vi "Lectura OSA (1).vi"() -> ()   [LabVIEW 2014]
panel:
  out "Read Data":string
  out "Respuesta OSA":string
  out "error out":errorcluster
  out "Array Data":dbl[](array[numeric]) format="%.5e"
  in  "Get data":bool
  in  "Send":bool
  out "Espectro":cluster{dbl[], dbl[]}(graph)
  out "?":bool
  in  "Sweep repeat":bool
  in  "Blank/Disp":bool=TRUE
  in  "?":bool
  in  "Stop":dbl=1570.0
  in  "Start":dbl=1470.0
  in  "Atributo":i32(listbox)
  in  "Trace":i32(listbox)
  in  "Preconfigurar":bool
  in  "Puerto":refnum<visa-resource-name>
  # "Sí"
  # "No"
  # "Span"
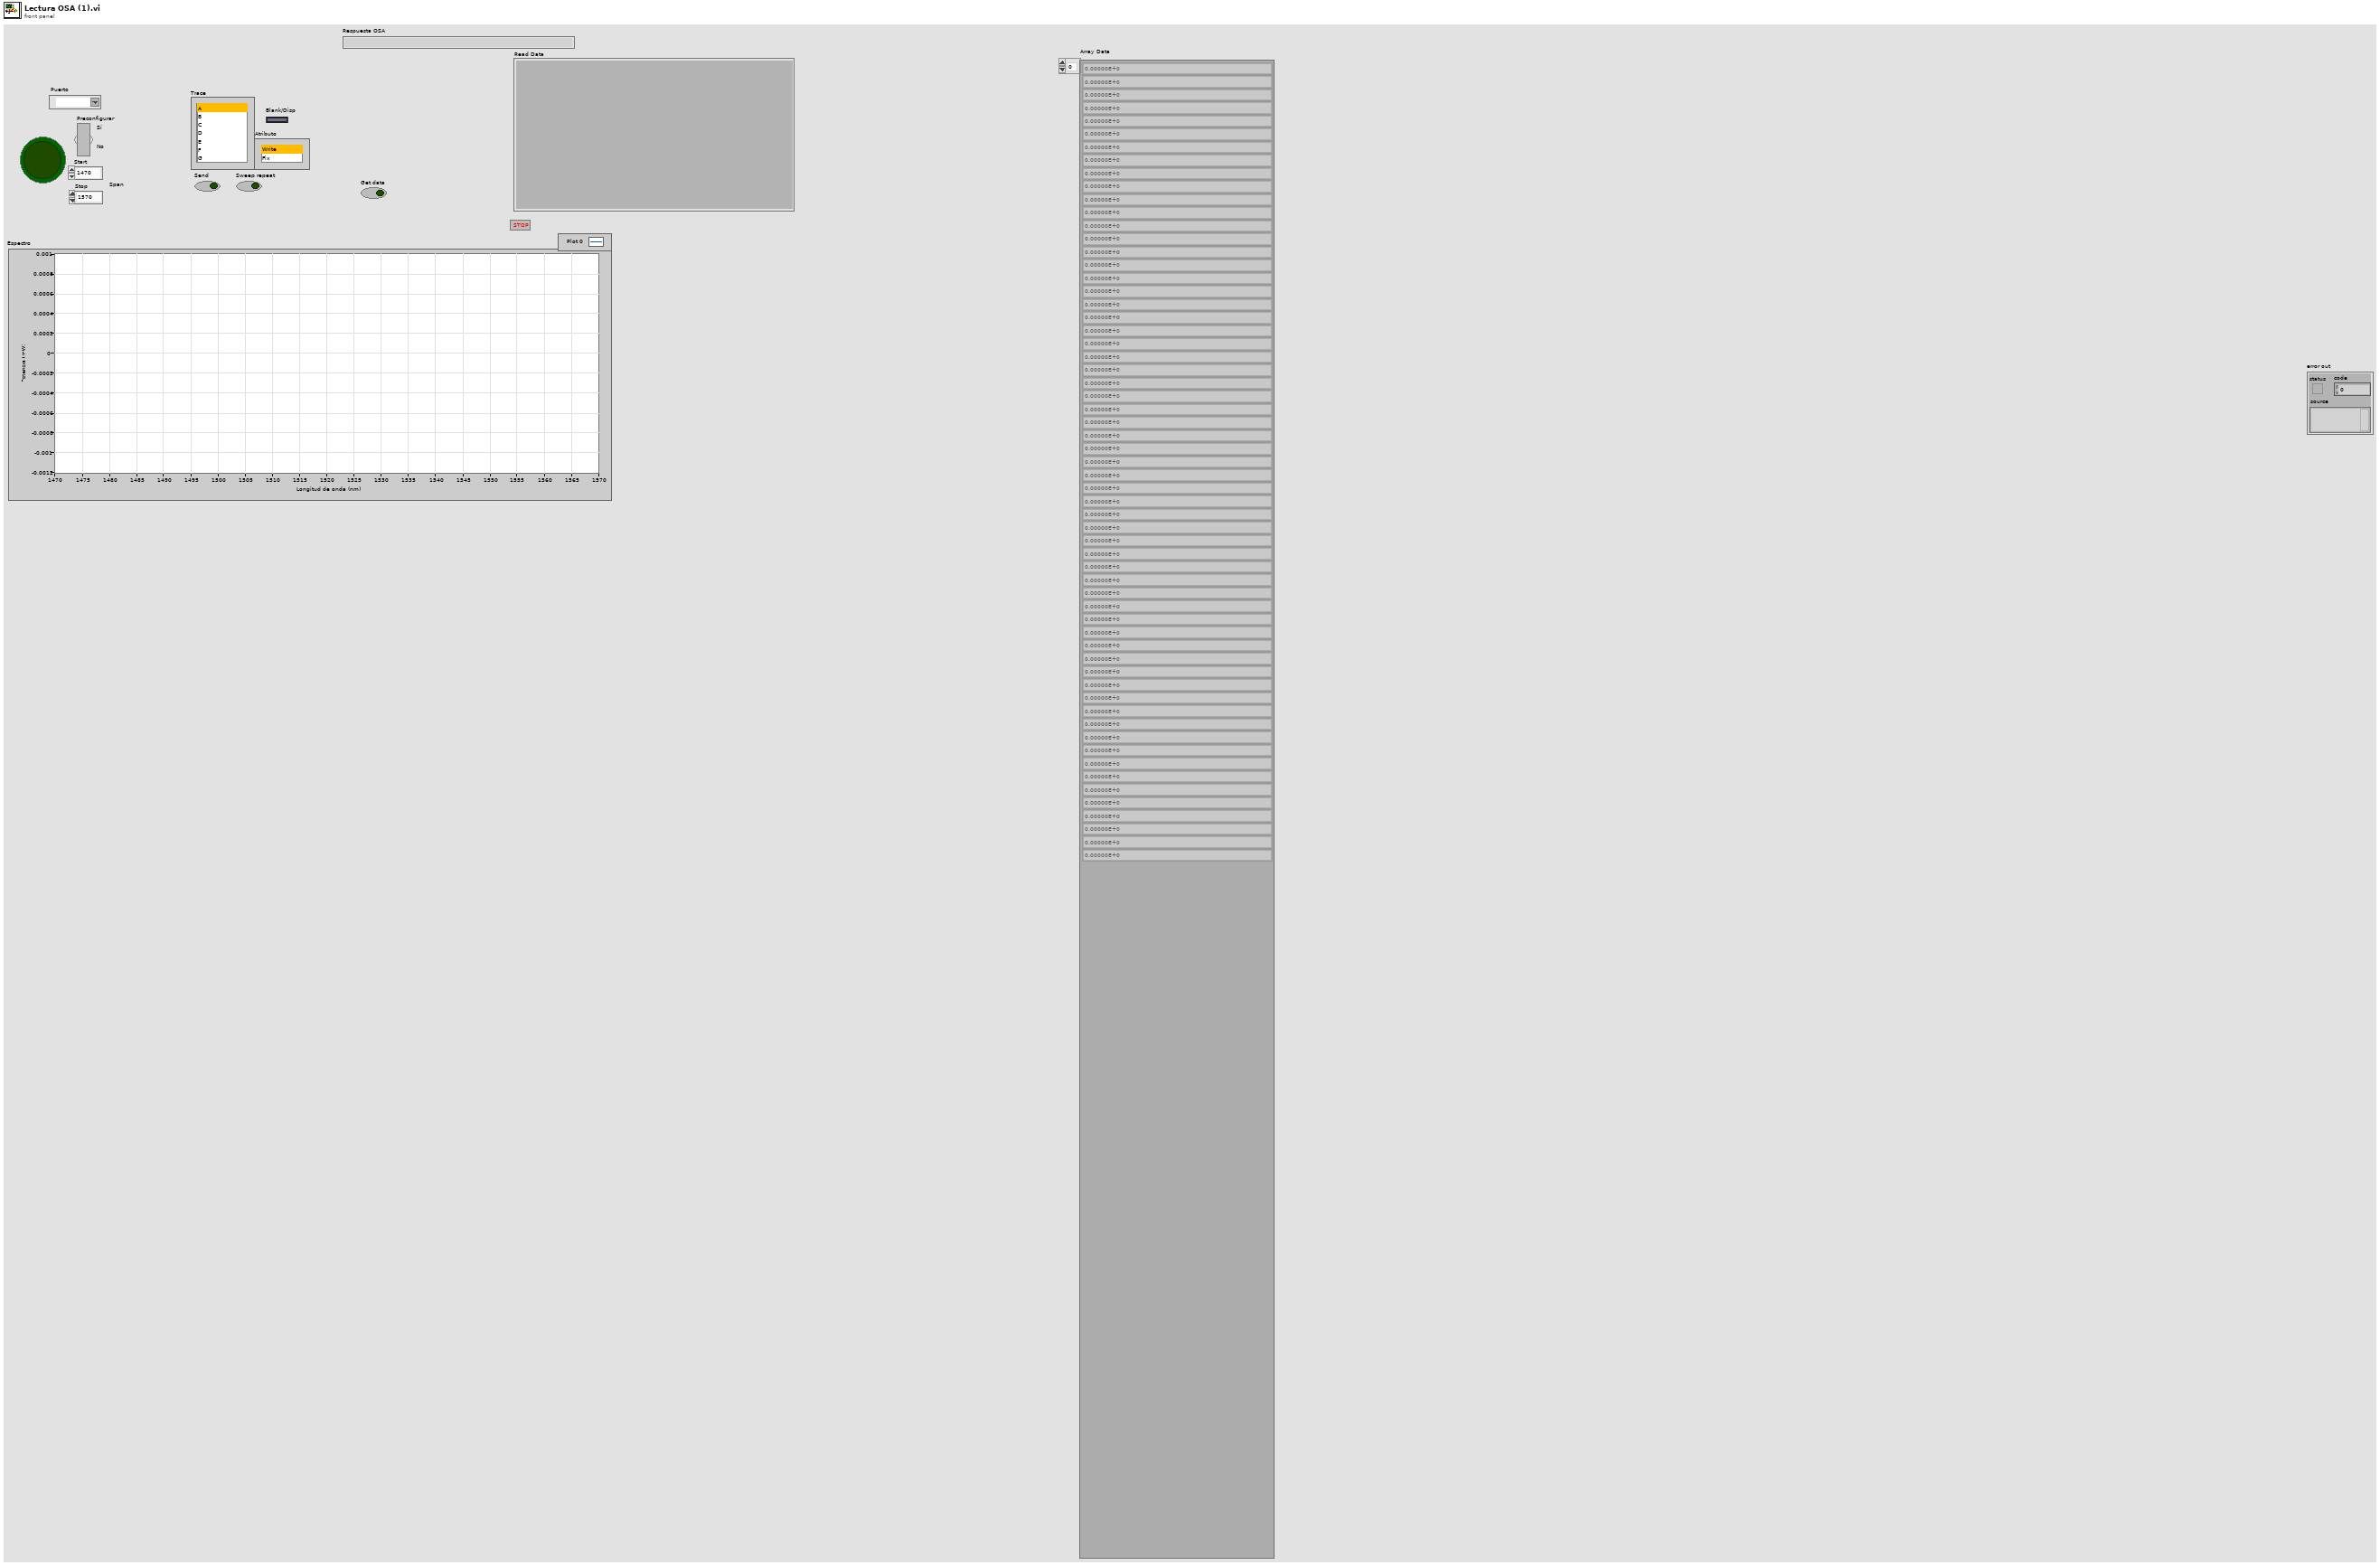
[diagram p1: front panel]
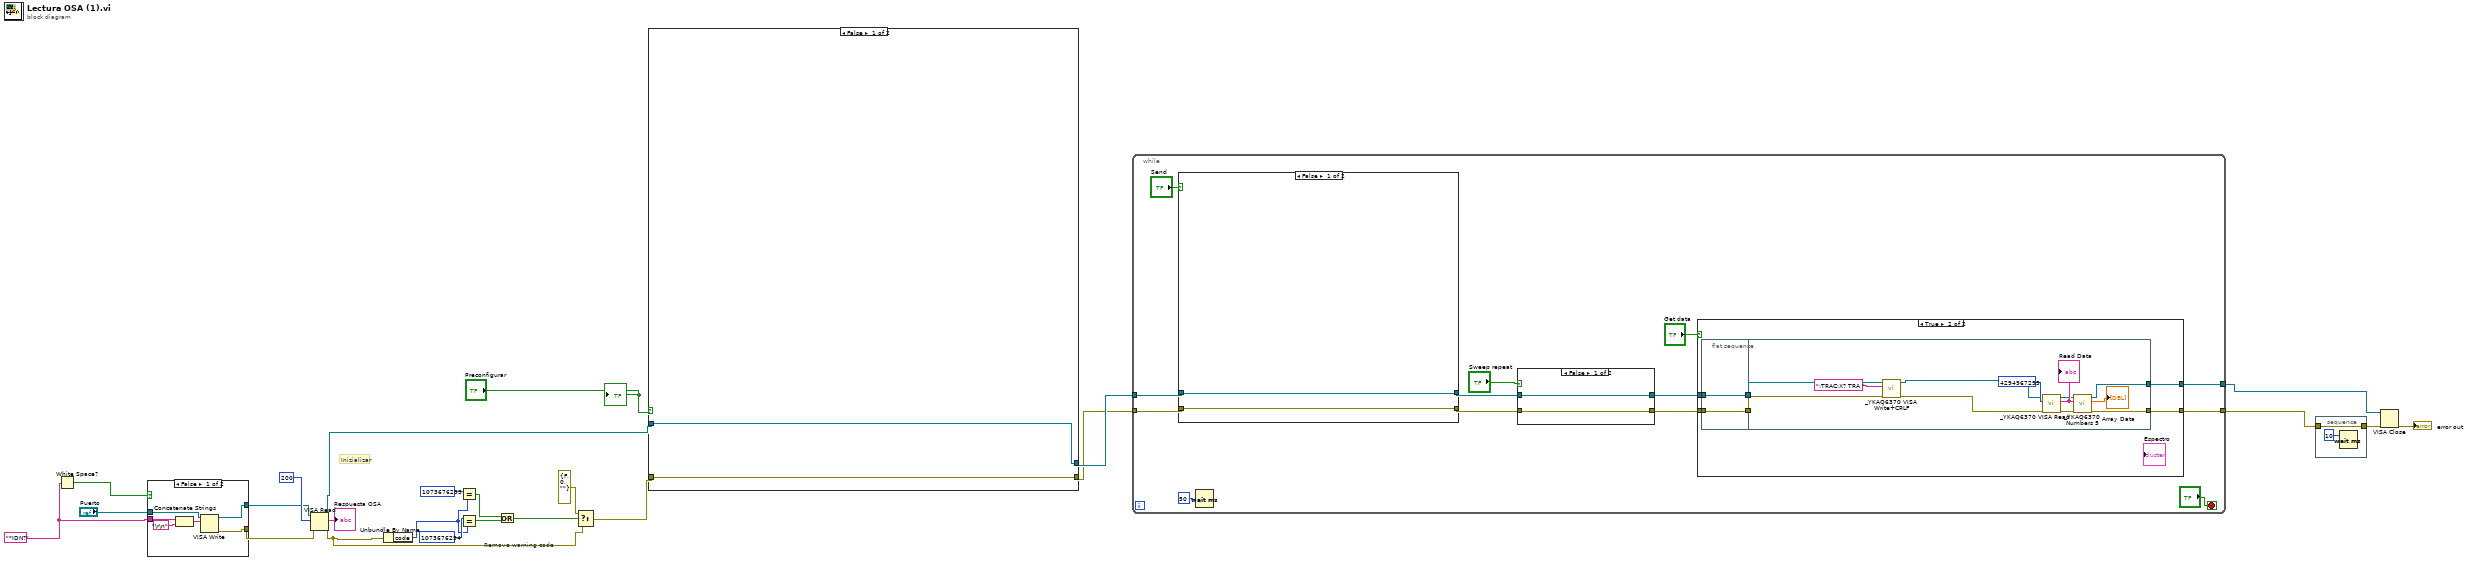
[diagram p0: block diagram]
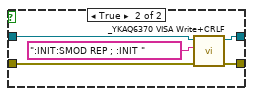
[diagram p3: hidden frame]
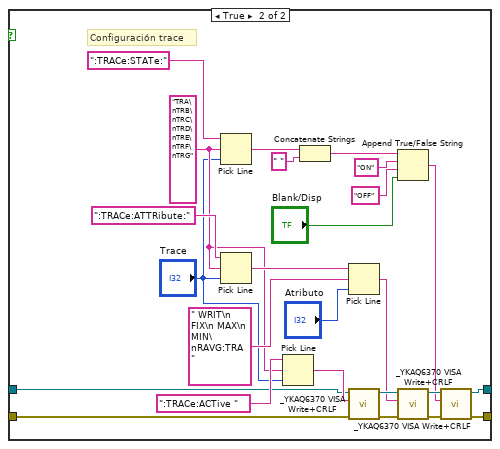
[diagram p4: hidden frame]
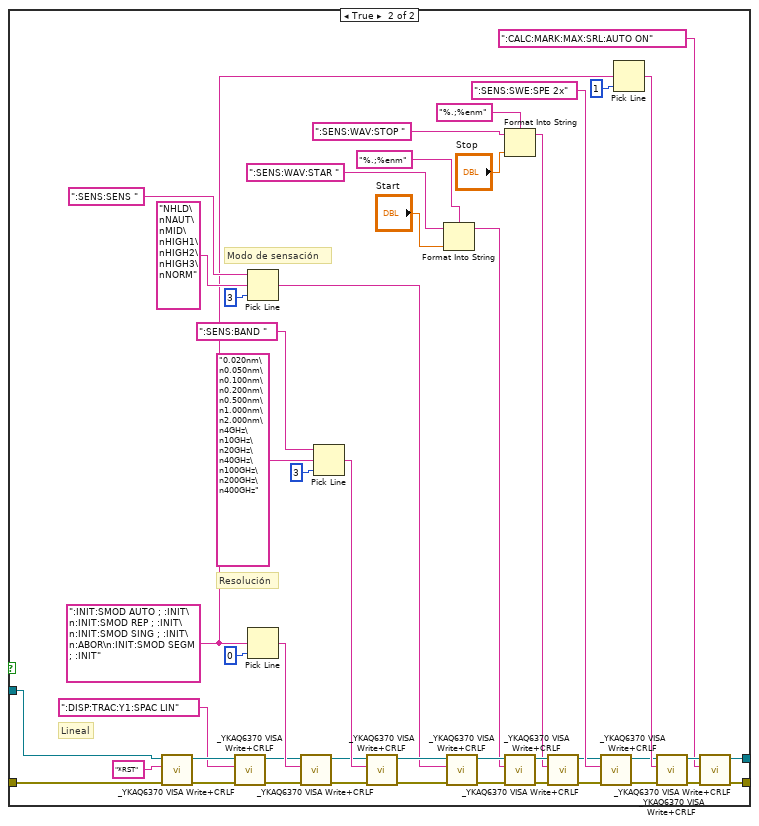
[diagram p5: hidden frame]
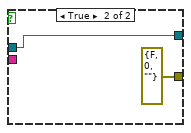
[diagram p6: hidden frame]
diagram:
  w22 = "*IDN?" ("Strings (empty)")
  # "Inizializar"
  # "Remove warning code"
  n1 = White Space?(1:w22) -> (0:w23:bool)
  n2 = case shown="False" w23 {
    tunnel: "Puerto" -> [w28 w32]
    tunnel: [w27 w32] -> w12
    tunnel: w22 -> [w26 _]
    tunnel: [w25 errorcluster {"status"=FALSE, "code"=0, "source"=""} ("error out")] -> w11
    frame False {
      n3 = Concatenate Strings(w26, "\r\n") -> (w29:string)
      n4 = VISA Write(VISA resource name=w28, write buffer=w29) -> (VISA resource name out=w27:refnum<visa-resource-name>, error out=w25:errorcluster)  [unwired: 1 in, 1 out]
    }
    frame True {
    }
  }
  n5 = VISA Read(VISA resource name=w12, byte count=u32 200 ("Byte Count (0)"), error in (no error)=w11) -> (VISA resource name out=w10:refnum<visa-resource-name>, read buffer=→"Respuesta OSA":string, error out=w19:errorcluster)  [unwired: 1 out]
  n6 = Unbundle By Name(w19) -> ("code"=w16:i32)
  n7 = Equal?(x=1073676293, y=w16) -> (x = y?=w15:bool)
  n8 = Equal?(x=1073676294, y=w16) -> (x = y?=w14:bool)
  n9 = Or(x=w15, y=w14) -> (x .or. y?=w13:bool)
  n10 = Select(t=errorcluster {"status"=FALSE, "code"=0, "source"=""}, s=w13, f=w19) -> (s? t:f=w9:errorcluster)
  n11 = case shown="False" "Preconfigurar" {
    tunnel: w10 -> [w34 w80]
    tunnel: w9 -> [w33 w79]
    tunnel: [w34 w39] -> w8
    tunnel: [w33 w38] -> w7
    frame False {
    }
    frame True {
      w50 = ":INIT:SMOD AUTO ; :INIT\n:INIT:SMOD REP ; :INIT\n:INIT:SMOD SING ; :INIT\n:ABOR\n:INIT:SMOD SEGM ; :INIT"
      # "Lineal"
      # "Modo de sensación"
      # "Resolución"
      n12 = call <instrlib>:"_YKAQ6370 VISA Write+CRLF.vi"("error in (no error)"=w79, "Strings (empty)"="*RST", "VISA resource name"=w80) -> ("error out"=w45:errorcluster, "VISA resource name out"=w46:refnum<visa-resource-name>)  [unwired: 7 in]
      n13 = call <instrlib>:"_YKAQ6370 VISA Write+CRLF.vi"("error in (no error)"=w45, "Strings (empty)"=":DISP:TRAC:Y1:SPAC LIN", "VISA resource name"=w46) -> ("error out"=w42:errorcluster, "VISA resource name out"=w43:refnum<visa-resource-name>)  [unwired: 7 in]
      n14 = Pick Line(string ("")=":SENS:SENS ", multi-line string="NHLD\nNAUT\nMID\nHIGH1\nHIGH2\nHIGH3\nNORM", line index=3) -> (output string=w72:string)
      n15 = Pick Line(multi-line string=w50, line index=0) -> (output string=w54:string)  [unwired: 1 in]
      n16 = call <instrlib>:"_YKAQ6370 VISA Write+CRLF.vi"("error in (no error)"=w42, "Strings (empty)"=w54, "VISA resource name"=w43) -> ("error out"=w55:errorcluster, "VISA resource name out"=w56:refnum<visa-resource-name>)  [unwired: 7 in]
      n17 = Pick Line(string ("")=":SENS:BAND ", multi-line string="0.020nm\n0.050nm\n0.100nm\n0.200nm\n0.500nm\n1.000nm\n2.000nm\n4GHz\n10GHz\n20GHz\n40GHz\n100GHz\n200GHz\n400GHz", line index=3) -> (output string=w67:string)
      n18 = call <instrlib>:"_YKAQ6370 VISA Write+CRLF.vi"("error in (no error)"=w55, "Strings (empty)"=w67, "VISA resource name"=w56) -> ("error out"=w76:errorcluster, "VISA resource name out"=w75:refnum<visa-resource-name>)  [unwired: 7 in]
      n19 = Format Into String(format string="%.;%enm", initial string=":SENS:WAV:STAR ", "Start") -> (resulting string=w61:string)  [unwired: 1 in, 1 out]
      n20 = call <instrlib>:"_YKAQ6370 VISA Write+CRLF.vi"("error in (no error)"=w76, "Strings (empty)"=w72, "VISA resource name"=w75) -> ("error out"=w77:errorcluster, "VISA resource name out"=w78:refnum<visa-resource-name>)  [unwired: 7 in]
      n21 = Format Into String(format string="%.;%enm", initial string=":SENS:WAV:STOP ", "Stop") -> (resulting string=w58:string)  [unwired: 1 in, 1 out]
      n22 = call <instrlib>:"_YKAQ6370 VISA Write+CRLF.vi"("error in (no error)"=w77, "Strings (empty)"=w61, "VISA resource name"=w78) -> ("error out"=w65:errorcluster, "VISA resource name out"=w66:refnum<visa-resource-name>)  [unwired: 7 in]
      n23 = call <instrlib>:"_YKAQ6370 VISA Write+CRLF.vi"("error in (no error)"=w65, "Strings (empty)"=w58, "VISA resource name"=w66) -> ("error out"=w40:errorcluster, "VISA resource name out"=w41:refnum<visa-resource-name>)  [unwired: 7 in]
      n24 = call <instrlib>:"_YKAQ6370 VISA Write+CRLF.vi"("error in (no error)"=w40, "Strings (empty)"=":SENS:SWE:SPE 2x", "VISA resource name"=w41) -> ("error out"=w48:errorcluster, "VISA resource name out"=w49:refnum<visa-resource-name>)  [unwired: 7 in]
      n25 = Pick Line(multi-line string=w50, line index=1) -> (output string=w51:string)  [unwired: 1 in]
      n26 = call <instrlib>:"_YKAQ6370 VISA Write+CRLF.vi"("error in (no error)"=w48, "Strings (empty)"=w51, "VISA resource name"=w49) -> ("error out"=w36:errorcluster, "VISA resource name out"=w37:refnum<visa-resource-name>)  [unwired: 7 in]
      n27 = call <instrlib>:"_YKAQ6370 VISA Write+CRLF.vi"("error in (no error)"=w36, "Strings (empty)"=":CALC:MARK:MAX:SRL:AUTO ON", "VISA resource name"=w37) -> ("error out"=w38:errorcluster, "VISA resource name out"=w39:refnum<visa-resource-name>)  [unwired: 7 in]
    }
  }
  n28 = while {
    tunnel: w8 -> [w94]
    tunnel: w7 -> [w93]
    tunnel: [w83] -> w2
    tunnel: [w82] -> w3
    stop <- "?" stop-if-true
    n29 = case shown="False" "Send" {
      tunnel: w94 -> [w125 w131]
      tunnel: w93 -> [w124 w130]
      tunnel: [w125 w128] -> w91
      tunnel: [w124 w127] -> w90
      frame False {
      }
      frame True {
        w133 = "TRA\nTRB\nTRC\nTRD\nTRE\nTRF\nTRG"
        # "Configuración trace"
        n30 = Pick Line(string ("")=":TRACe:STATe:", multi-line string=w133, line index="Trace") -> (output string=w134:string)
        n31 = Pick Line(string ("")=":TRACe:ATTRibute:", multi-line string=w133, line index="Trace") -> (output string=w139:string)
        n32 = Pick Line(string ("")=":TRACe:ACTive ", multi-line string=w133, line index="Trace") -> (output string=w135:string)
        n33 = Concatenate Strings(w134, " " ("string")) -> (w137:string)
        n34 = Pick Line(string ("")=w139, multi-line string=" WRIT\n FIX\n MAX\n MIN\nRAVG:TRA ", line index="Atributo") -> (output string=w138:string)
        n35 = call <instrlib>:"_YKAQ6370 VISA Write+CRLF.vi"("error in (no error)"=w130, "Strings (empty)"=w135, "VISA resource name"=w131) -> ("error out"=w147:errorcluster, "VISA resource name out"=w146:refnum<visa-resource-name>)  [unwired: 7 in]
        n36 = Append True/False String(1:"Blank/Disp", 2:"OFF", 3:"ON", 4:w137) -> (0:w143:string)
        n37 = call <instrlib>:"_YKAQ6370 VISA Write+CRLF.vi"("error in (no error)"=w147, "Strings (empty)"=w138, "VISA resource name"=w146) -> ("error out"=w144:errorcluster, "VISA resource name out"=w145:refnum<visa-resource-name>)  [unwired: 7 in]
        n38 = call <instrlib>:"_YKAQ6370 VISA Write+CRLF.vi"("error in (no error)"=w144, "Strings (empty)"=w143, "VISA resource name"=w145) -> ("error out"=w127:errorcluster, "VISA resource name out"=w128:refnum<visa-resource-name>)  [unwired: 7 in]
      }
    }
    n39 = Wait (ms)(milliseconds to wait=u32 50) -> ()  [unwired: 1 out]
    n40 = case shown="False" "Sweep repeat" {
      tunnel: w91 -> [w118 w123]
      tunnel: w90 -> [w117 w122]
      tunnel: [w118 w120] -> w86
      tunnel: [w117 w119] -> w85
      frame False {
      }
      frame True {
        n41 = call <instrlib>:"_YKAQ6370 VISA Write+CRLF.vi"("error in (no error)"=w122, "Strings (empty)"=":INIT:SMOD REP ; :INIT ", "VISA resource name"=w123) -> ("error out"=w119:errorcluster, "VISA resource name out"=w120:refnum<visa-resource-name>)  [unwired: 7 in]
      }
    }
    n42 = case shown="True" "Get data" {
      tunnel: w86 -> [w95 w102]
      tunnel: w85 -> [w96 w101]
      tunnel: [w96 w100] -> w83
      tunnel: [w95 w97] -> w82
      frame False {
      }
      frame True {
        n43 = flat-sequence {
          tunnel: w102 -> [w104]
          tunnel: w101 -> [w103]
          tunnel: [w104] -> w99
          tunnel: [w103] -> w98
          tunnel: [w111] -> w100
          tunnel: [w110] -> w97
          tunnel: w99 -> [w106]
          tunnel: w98 -> [w105]
          frame #0 {
          }
          frame #1 {
            n44 = call <instrlib>:"_YKAQ6370 VISA Write+CRLF.vi"("error in (no error)"=w105, "Strings (empty)"=":TRAC:X? TRA ", "VISA resource name"=w106) -> ("error out"=w108:errorcluster, "VISA resource name out"=w109:refnum<visa-resource-name>)  [unwired: 7 in]
            n45 = call "_YKAQ6370 VISA Read.vi"("error in (no error)"=w108, "Byte Count (0)"=u32 4294967295, "VISA resource name"=w109) -> ("error out"=w112:errorcluster, "Read Data"=w115:string, "VISA resource name out"=w113:refnum<visa-resource-name>)  [unwired: 5 in, 1 out]
            "Read Data" <- w115
            n46 = call <instrlib>:"_YKAQ6370 Numbers 5.vi"("error in (no error)"=w112, "String"=w115, "VISA resource name"=w113) -> ("error out"=w111:errorcluster, "Array Data"=→"Array Data":dbl[], "VISA resource name out"=w110:refnum<visa-resource-name>)  [unwired: 6 in]
          }
        }
      }
    }
  }
  n47 = stacked-sequence {
    tunnel: [w151] -> w4
    tunnel: w2 -> [w151]
    frame #0 {
      n48 = Wait (ms)(milliseconds to wait=u32 10) -> ()  [unwired: 1 out]
    }
  }
  n49 = VISA Close(VISA resource name=w3, error in (no error)=w4) -> (error out=→"error out":errorcluster)
  "?" <- "Preconfigurar"
